vi "TestForceGraph 2.vi"() -> ()   [LabVIEW 2017]
panel:
  in  "Full Angle":dbl=6.0
  in  "Full Angle Tolerance":dbl=3.0
  in  "Peak Force Tolerance":dbl=3.0
  in  "Peak Force":dbl=4.0
  in  "Force Annotation":bool=TRUE
  in  "Expand":bool=TRUE
  in  "Auto":bool
  in  "First Touch":bool
  in  "Path":path
  in  "Filenames":string[](array[string])
  in  "FileType":string(combo)="DL"
  out "Graph":cluster{"Y":dbl[], "Y":dbl[]}[](graph)
  # "RL\nUp/Down"
  # "RR\nUp/Down"
  # "FL\nUp/Down"
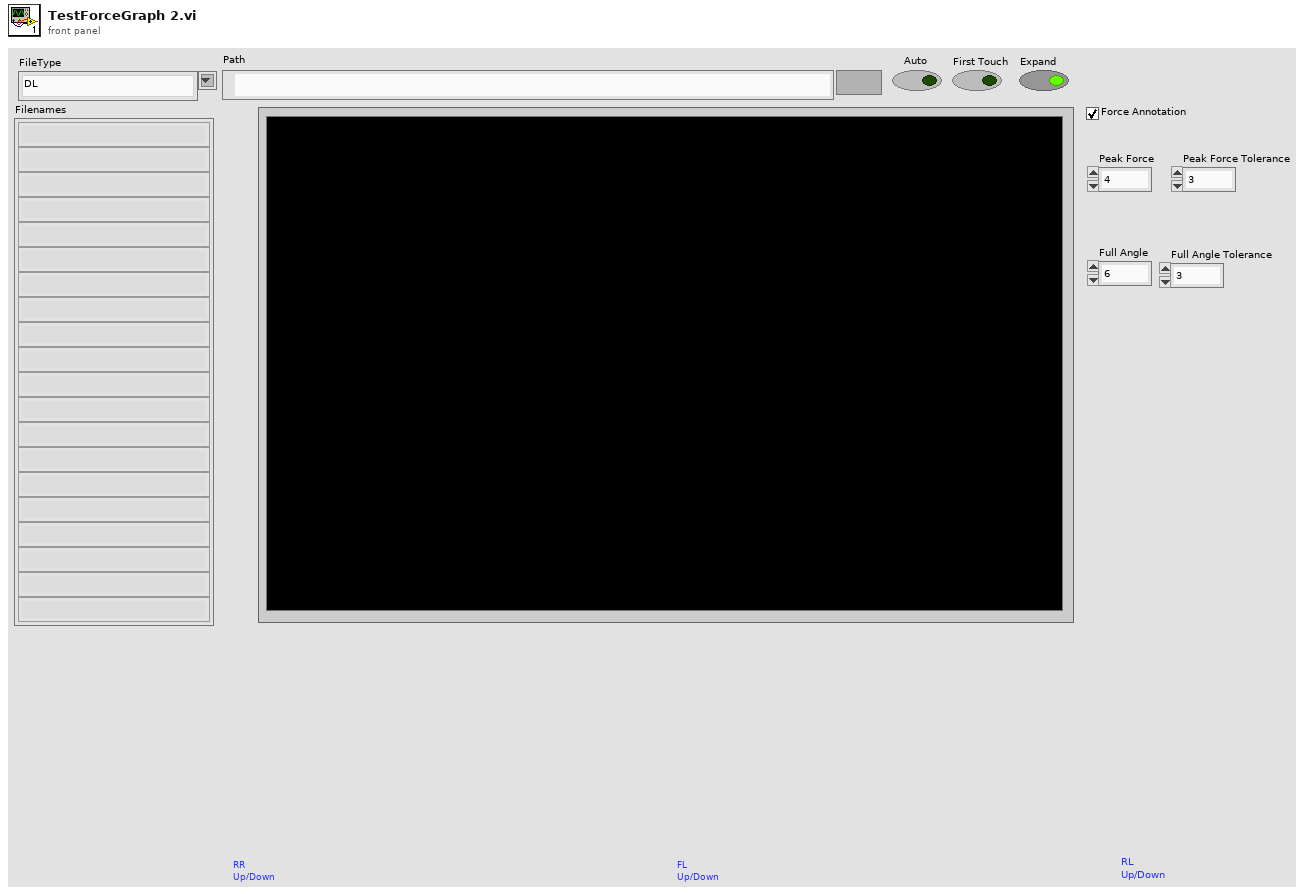
[diagram p1: front panel]
types:
  T1 = cluster{"DownMax":u16, "DownMin":u16, "UpMax":u16, "UpMin":u16}
  T2 = cluster{"Peak_Force":dbl, "Peak_Force_Tolerance":dbl, "Full_Angle":dbl, "Full_Angle_Tolerance":dbl}
  T3 = cluster{"Angle Data":dbl[], "Force Data":dbl[], "Volt Data 1":dbl[], "Volt Data 2":dbl[]}
  T4 = cluster{"Angle Data":dbl[], "Force Data 1":dbl[], "Force Data 2":dbl[], "Volt Data 1":dbl[], "Volt Data 2":dbl[]}
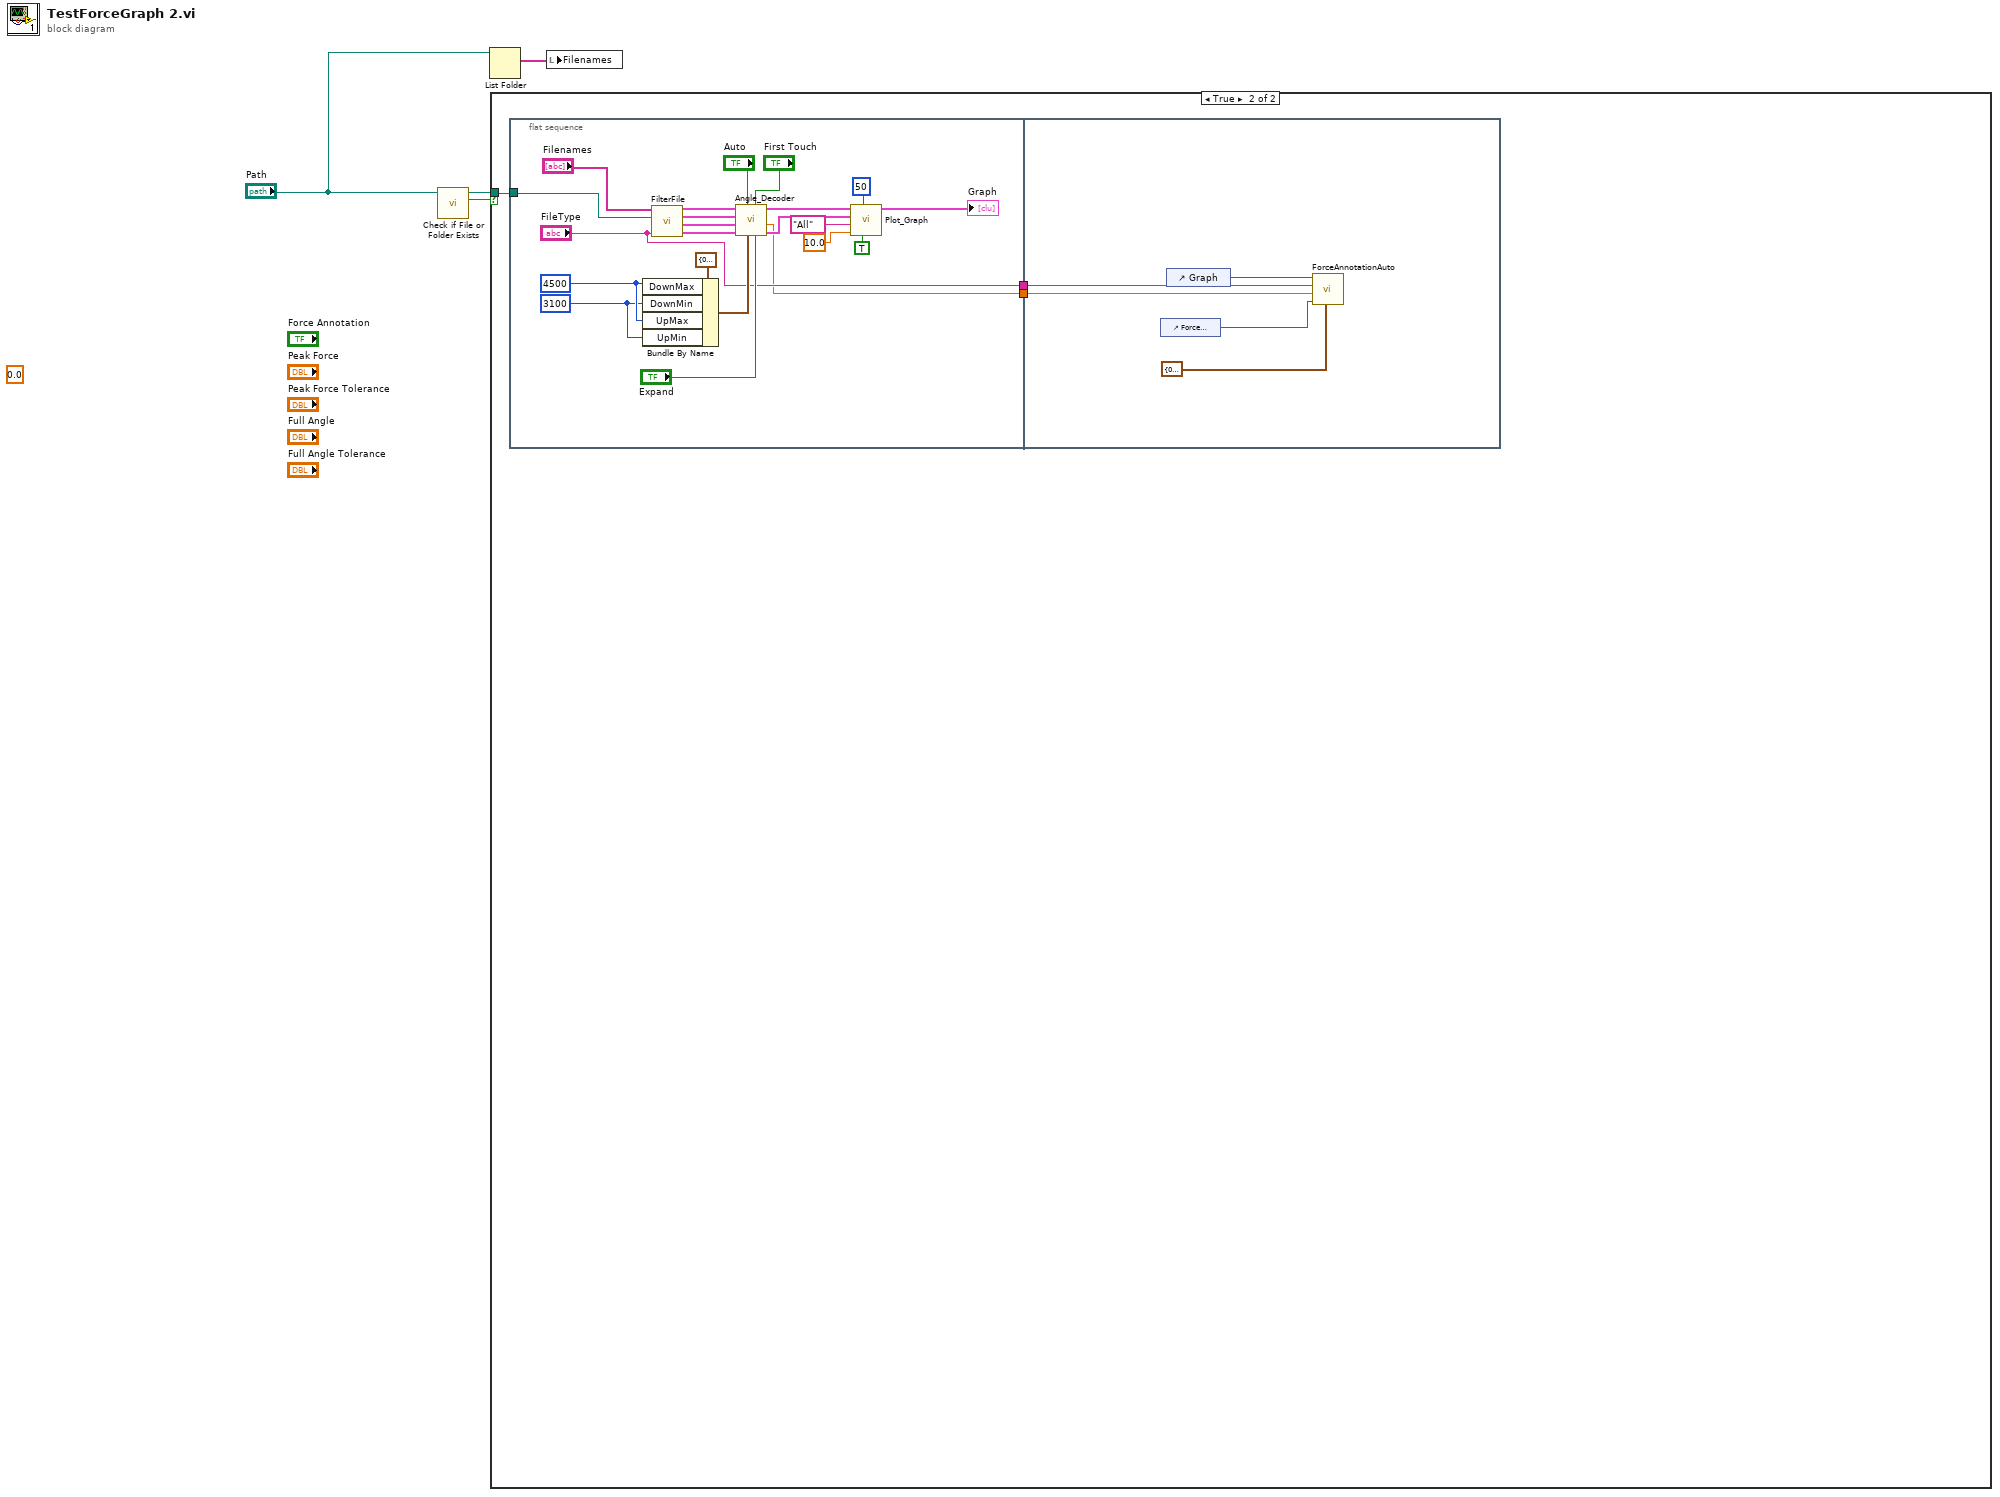
[diagram p0: block diagram]
diagram:
  (unwired) 0.0 ("ForceMemory")
  n1 = call <vilib>:"Check if File or Folder Exists.vi"("path"="Path") -> ("file or folder exists?"=w3:bool, "dup path"=w1:path)  [unwired: 8 in, 1 out]
  n2 = List Folder(path="Path") -> (filenames=w4:string[])  [unwired: 3 in, 3 out]
  n3 = case shown="True" w3 {
    tunnel: w1 -> [_ w7]
    frame False {
    }
    frame True {
      n4 = flat-sequence {
        tunnel: w7 -> [w20]
        tunnel: ["FileType"] -> w6
        tunnel: [w8] -> w5
        tunnel: w6 -> [w33]
        tunnel: w5 -> [w30]
        frame #0 {
          w13 = u16 3100
          w14 = u16 4500
          n5 = Bundle By Name(cluster=T1 {"DownMax"=0, "DownMin"=0, "UpMax"=0, "UpMin"=0} ("AngleUpDown"), "DownMax"=w14, "DownMin"=w13, "UpMax"=w14, "UpMin"=w13) -> (w22:T1)
          n6 = call "FilterFile.vi"("FileType"="FileType", "Path"=w20, "Filenames"="Filenames") -> ("RW_Up"=w29:T3, "FW_Up"=w18:T3, "RW_Down"=w28:T3, "FW_Down"=w19:T3)  [unwired: 3 in, 2 out]
          n7 = call "Angle_Decoder.vi"("Expand"="Expand", "Find Fist Touch"="First Touch", "AngleUpDown"=w22, "Auto/Manual"="Auto", "Analog RW Up"=w29, "Analog FW Up"=w18, "Analog RW Down"=w28, "Analog FW Down"=w19) -> ("Analog RW D/U"=w16:T4, "Last Angle"=w8:dbl, "Analog FW D/U"=w17:T4)  [unwired: 1 in]
          n8 = call "Plot_Graph.vi"("EnableSmooth"=TRUE, "FillZeroFirstSignal"=50, "VoltDevider"=10.0, "Channel"="All", "Analog RW In"=w16, "Analog FW In"=w17) -> ("XY Graph"=→"Graph":cluster{"Angle Data":dbl[], "Array":dbl[]}[])  [unwired: 5 in]
        }
        frame #1 {
          n9 = control-ref of="Force Annotation"() -> (w32:refnum<vi>)
          n10 = control-ref of="Graph"() -> (w34:refnum<vi>)
          n11 = call "ForceAnnotationAuto.vi"("SpectConfig"=T2 {"Peak_Force"=0.0, "Peak_Force_Tolerance"=0.0, "Full_Angle"=0.0, "Full_Angle_Tolerance"=0.0}, "EN"=w32, "LastAngle"=w30, "Test Name"=w33, "Graph"=w34) -> ()  [unwired: 7 in]
        }
      }
    }
  }
  n12 = local write "Filenames"(w4) -> ()
